vi "IMICSDK_GUI.vi"() -> ()   [LabVIEW 2011]
uses:
  <vilib>/Utility/cursorutil.llb/Set Cursor (Icon Pict).vi
panel:
  in  "Cluster":T1
  in  "resP":dbl=0.001
  in  "res":dbl=0.1
  in  "close at end":bool
  out "Status":T2(ring)
  in  "stop":bool
  in  "X":dbl(slide) min=0.0 scale=10.0..12.5
  in  "Y":dbl(slide) min=0.0 scale=0.0..22.0
  in  "Piezo":dbl(slide) step=0.005 scale=0.0..0.25 scale format="%#.4g"
  in  "Objektive":u16(ring) items=["Obj1 10x", "Obj2", "Obj3", "Obj4"]
  in  "FilterSchieber 1":u16(ring) items=["Filter 1", "Filter 2", "Filter 3"]
  in  "Z":dbl(slide) min=0.0 max=20.0 step=0.01 scale=18.0..20.0
  in  "handle":u64
  in  "comport":string="com1"
  # "xyz res."
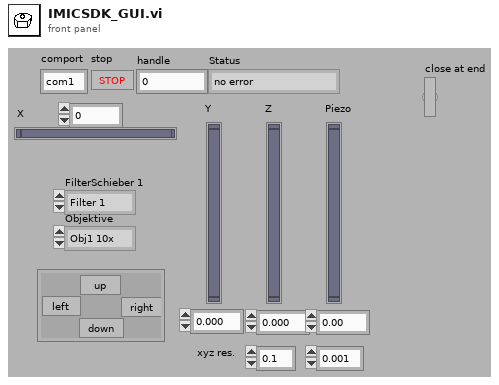
[diagram p1: front panel]
types:
  T1 = cluster{"up":bool, "left":bool, "right":bool, "down":bool}
  T2 = enum16{"no error", "missing axis", "missing Z axis", "missing Filter", "iMic not initialized", "no property", "wrong handle", "protocol not finished", "user parameter to long (>32 bits)", "no user parameter handle", "failed to open comport", "failed to initialize"}
  T3 = typedef "eventvkey.ctl" = enum16{"ASCII", "Enter", "Return", "Shift", "Ctrl", "Alt", "Cmd", "Opt", "Caps", "NumLock", "Clear", "Break", "Up", "Down", "Left", "Right", "Insert", "Delete", "Home", "End", "PageUp", "PageDown", "Escape", "Help", "Pause", "ScrollLock", "F1", "F2", "F3", "F4", "F5", "F6", "F7", "F8", "F9", "F10", "F11", "F12", "F13", "F14", "F15", "F16", "F17", "F18", "F19", "F20", "F21", "F22", "F23", "F24", "Play", "VolumeUp", "VolumeDown", "Mute", "Two Byte Char"}
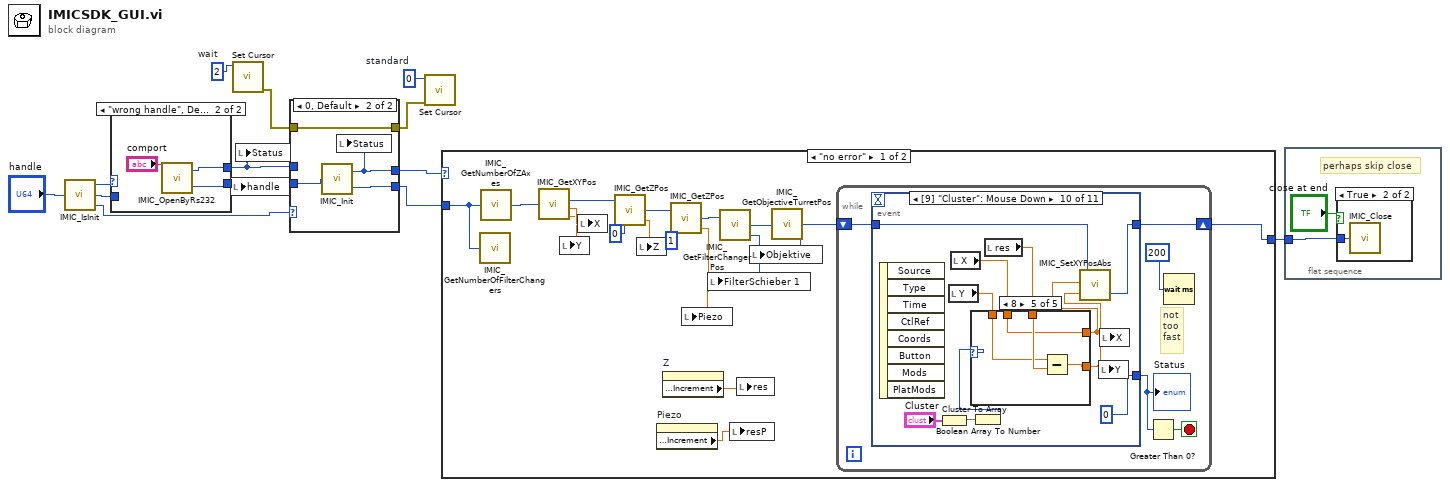
[diagram p0: block diagram]
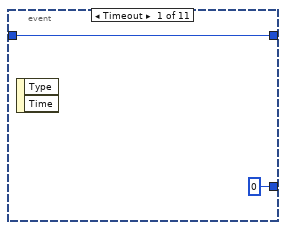
[diagram p5: hidden frame]
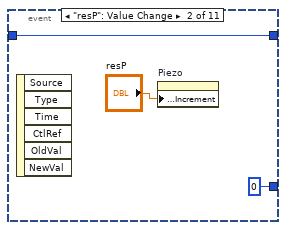
[diagram p6: hidden frame]
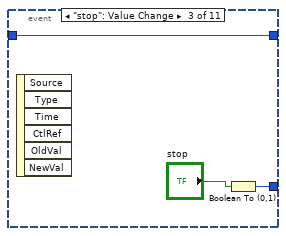
[diagram p7: hidden frame]
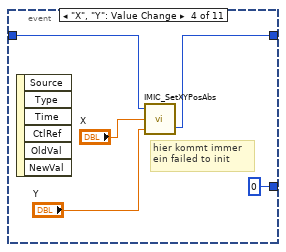
[diagram p8: hidden frame]
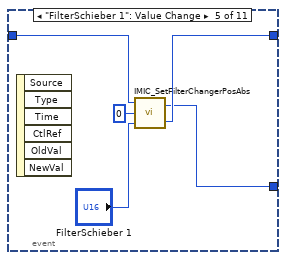
[diagram p9: hidden frame]
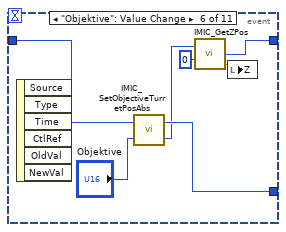
[diagram p10: hidden frame]
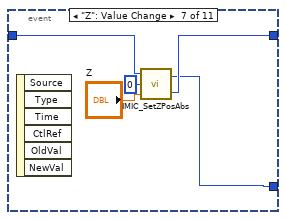
[diagram p11: hidden frame]
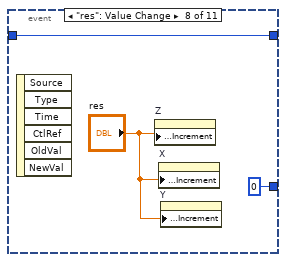
[diagram p12: hidden frame]
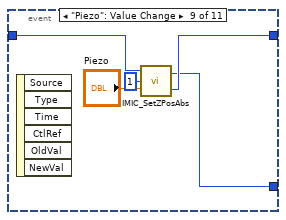
[diagram p13: hidden frame]
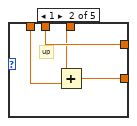
[diagram p15: hidden frame]
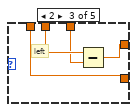
[diagram p16: hidden frame]
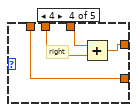
[diagram p17: hidden frame]
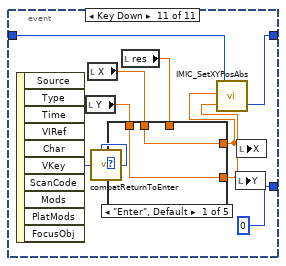
[diagram p18: hidden frame]
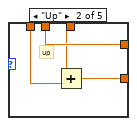
[diagram p19: hidden frame]
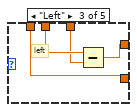
[diagram p20: hidden frame]
diagram:
  w8 = u16 2  # wait
  w9 = u16 0  # standard
  n1 = call "IMIC_IsInit.vi"("handle"="handle") -> ("output param"=w11:T2, "handle out"=w10:u64, "bool"=w3:i8)
  n2 = case shown="\"wrong handle\", Default" w11 {
    selector: w11 -> [w14 _]
    tunnel: [w15 w17] -> w2
    tunnel: w10 -> [w15 _]
    tunnel: [w14 w16] -> w1
    frame "no error" {
    }
    frame "wrong handle", Default {
      n3 = call "IMIC_OpenByRs232.vi"("comport"="comport") -> ("output param"=w16:T2, "handle out"=w17:u64)
    }
  }
  n4 = local write "handle"(w2) -> ()
  n5 = call-poly <vilib>:"Set Cursor.vi"("icon"=w8) -> ("error out"=w7:errorcluster)  [unwired: 9 in, 1 out]
  n6 = local write "Status"(w1) -> ()
  n7 = case shown="0, Default" w3 {
    tunnel: w7 -> [w19 w25]
    tunnel: [w19 w25] -> w6
    tunnel: w2 -> [w21 w24]
    tunnel: [w20 w22] -> w4
    tunnel: [w21 w23] -> w5
    tunnel: w1 -> [w20 _]
    frame 1 {
    }
    frame 0, Default {
      n8 = call "IMIC_Init.vi"("handle"=w24) -> ("output param"=w22:T2, "handle out"=w23:u64)
      n9 = local write "Status"(w22) -> ()
    }
  }
  n10 = call-poly <vilib>:"Set Cursor.vi"("error in (no error)"=w6, "icon"=w9) -> ()  [unwired: 8 in, 2 out]
  n11 = case shown="\"no error\"" w4 {
    tunnel: [w30 w144] -> w13
    tunnel: w5 -> [w29 w144]
    frame "no error" {
      n12 = call "IMIC_GetNumberOfFilterChangers.vi"("handle"=w29) -> ()  [unwired: 3 out]
      n13 = call "IMIC_GetNumberOfZAxes.vi"("handle"=w29) -> ("handle out"=w39:u64)  [unwired: 2 out]
      n14 = call "IMIC_GetXYPos.vi"("handle"=w39) -> ("handle out"=w35:u64, "xpos"=w37:dbl, "ypos"=w36:dbl)  [unwired: 1 out]
      n15 = local write "Y"(w36) -> ()
      n16 = local write "X"(w37) -> ()
      n17 = call "IMIC_GetZPos.vi"("handle"=w35, "index"=0) -> ("handle out"=w34:u64, "zpos"=w43:dbl)  [unwired: 1 out]
      n18 = local write "Z"(w43) -> ()
      n19 = property on="Piezo" class="Slide (strict)"() -> ("Data Entry Limits:Increment"=w27:dbl)  [unwired: 2 in, 2 out]
      n20 = property on="Z" class="Slide (strict)"() -> ("Data Entry Limits:Increment"=w28:dbl)  [unwired: 2 in, 2 out]
      n21 = call "IMIC_GetZPos.vi"("handle"=w34, "index"=1) -> ("handle out"=w33:u64, "zpos"=w26:dbl)  [unwired: 1 out]
      n22 = local write "Piezo"(w26) -> ()
      n23 = call "IMIC_GetFilterChangerPos.vi"("handle"=w33) -> ("handle out"=w32:u64, "Filter"=w42:i32)  [unwired: 1 in, 1 out]
      n24 = local write "FilterSchieber 1"(w42) -> ()
      n25 = local write "resP"(w27) -> ()
      n26 = local write "res"(w28) -> ()
      n27 = call "IMIC_GetObjectiveTurretPos.vi"("handle"=w32) -> ("handle out"=w31:u64, "Objective"=w41:i32)  [unwired: 1 out]
      n28 = local write "Objektive"(w41) -> ()
      n29 = while {
        shift-right: [w47] -> w30
        shift-left: w31 -> [w48]
        stop <- w44 stop-if-true
        # "not\ntoo\nfast"
        n30 = event shown="[9] \"Cluster\": Mouse Down" {
          selector: _ -> [_ _ _ _ _ _ _ _ _ _ _]
          dyn-events: _ -> [_ _ _ _ _ _ _ _ _ _ _]
          timeout: _ -> [_ _ _ _ _ _ _ _ _ _ _]
          tunnel: w48 -> [w50 w52 w56 w61 w64 w73 w76 w81 w85 w97 w125]
          tunnel: [w50 w52 w56 w60 w63 w68 w75 w81 w84 w88 w119] -> w47
          tunnel: [u16 0 ("output param") u16 0 ("output param") w54 u16 0 ("output param") w62 w71 w74 u16 0 ("output param") w83 0 0] -> w45
          event Timeout {
            n31 = event-data() -> ()  [unwired: 1 in, 2 out]
          }
          event "resP": Value Change {
            n32 = event-data() -> ()  [unwired: 1 in, 6 out]
            n33 = property on="Piezo" class="Slide (strict)"("Data Entry Limits:Increment"="resP") -> ()  [unwired: 2 in, 2 out]
          }
          event "stop": Value Change {
            n34 = event-data() -> ()  [unwired: 1 in, 6 out]
            n35 = Boolean To (0,1)(Boolean="stop") -> (0, 1=w54:i16)
          }
          event "X", "Y": Value Change {
            # "hier kommt immer\nein failed to init"
            n36 = event-data() -> ()  [unwired: 1 in, 6 out]
            n37 = call "IMIC_SetXYPosAbs.vi"("ypos"="Y", "xpos"="X", "handle"=w61) -> ("handle out"=w60:u64)  [unwired: 1 out]
          }
          event "FilterSchieber 1": Value Change {
            n38 = event-data() -> ()  [unwired: 1 in, 6 out]
            n39 = call "IMIC_SetFilterChangerPosAbs.vi"("Filter"="FilterSchieber 1", "index"=0, "handle"=w64) -> ("handle out"=w63:u64, "output param"=w62:T2)
          }
          event "Objektive": Value Change {
            n40 = event-data() -> ()  [unwired: 1 in, 6 out]
            n41 = call "IMIC_SetObjectiveTurretPosAbs.vi"("ObjectivePosAbs"="Objektive", "handle"=w73) -> ("handle out"=w69:u64, "output param"=w71:T2)
            n42 = call "IMIC_GetZPos.vi"("handle"=w69, "index"=0) -> ("handle out"=w68:u64, "zpos"=w67:dbl)  [unwired: 1 out]
            n43 = local write "Z"(w67) -> ()
          }
          event "Z": Value Change {
            n44 = event-data() -> ()  [unwired: 1 in, 6 out]
            n45 = call "IMIC_SetZPosAbs.vi"("zpos"="Z", "index"=0, "handle"=w76) -> ("handle out"=w75:u64, "output param"=w74:T2)
          }
          event "res": Value Change {
            n46 = event-data() -> ()  [unwired: 1 in, 6 out]
            n47 = property on="Z" class="Slide (strict)"("Data Entry Limits:Increment"="res") -> ()  [unwired: 2 in, 2 out]
            n48 = property on="X" class="Slide (strict)"("Data Entry Limits:Increment"="res") -> ()  [unwired: 2 in, 2 out]
            n49 = property on="Y" class="Slide (strict)"("Data Entry Limits:Increment"="res") -> ()  [unwired: 2 in, 2 out]
          }
          event "Piezo": Value Change {
            n50 = event-data() -> ()  [unwired: 1 in, 6 out]
            n51 = call "IMIC_SetZPosAbs.vi"("zpos"="Piezo", "index"=1, "handle"=w85) -> ("handle out"=w84:u64, "output param"=w83:T2)
          }
          event "Cluster": Mouse Down {
            n52 = event-data() -> ()  [unwired: 1 in, 8 out]
            n53 = Cluster To Array(cluster="Cluster") -> (array=w96:bool[])
            n54 = local read "Y"() -> (w91:dbl)
            n55 = local read "X"() -> (w92:dbl)
            n56 = Boolean Array To Number(Boolean array=w96) -> (number=w94:u32)
            n57 = local read "res"() -> (w93:dbl)
            n58 = case shown="8" w94 {
              tunnel: w93 -> [_ w101 w106 w110 w114]
              tunnel: w92 -> [w99 w103 w107 w109 w112]
              tunnel: w91 -> [w98 w102 w104 w108 w113]
              tunnel: [w99 w103 w105 w111 w112] -> w89
              tunnel: [w98 w100 w104 w108 w115] -> w90
              frame 0, Default {
              }
              frame 1 {
                # "up"
                n59 = Add(x=w101, y=w102) -> (x+y=w100:dbl)
              }
              frame 2 {
                # "left"
                n60 = Subtract(x=w107, y=w106) -> (x-y=w105:dbl)
              }
              frame 4 {
                # "right"
                n61 = Add(x=w110, y=w109) -> (x+y=w111:dbl)
              }
              frame 8 {
                n62 = Subtract(x=w113, y=w114) -> (x-y=w115:dbl)
              }
            }
            n63 = call "IMIC_SetXYPosAbs.vi"("ypos"=w90, "xpos"=w89, "handle"=w97) -> ("handle out"=w88:u64)  [unwired: 1 out]
            n64 = local write "Y"(w90) -> ()
            n65 = local write "X"(w89) -> ()
          }
          event Key Down {
            n66 = event-data() -> ("VKey"=w116:T3)  [unwired: 1 in, 9 out]
            n67 = local read "Y"() -> (w122:dbl)
            n68 = local read "X"() -> (w123:dbl)
            n69 = call <vilib>:"compatReturnToEnter.vi"("VKey"=w116) -> ("VKey"=w117:T3)
            n70 = local read "res"() -> (w124:dbl)
            n71 = case shown="\"Enter\", Default" w117 {
              tunnel: w124 -> [_ w129 w134 w138 w142]
              tunnel: w123 -> [w127 w131 w135 w137 w140]
              tunnel: w122 -> [w126 w130 w132 w136 w141]
              tunnel: [w127 w131 w133 w139 w140] -> w120
              tunnel: [w126 w128 w132 w136 w143] -> w121
              frame "Enter", Default {
              }
              frame "Up" {
                # "up"
                n72 = Add(x=w129, y=w130) -> (x+y=w128:dbl)
              }
              frame "Left" {
                # "left"
                n73 = Subtract(x=w135, y=w134) -> (x-y=w133:dbl)
              }
              frame "Right" {
                # "right"
                n74 = Add(x=w138, y=w137) -> (x+y=w139:dbl)
              }
              frame "Down" {
                n75 = Subtract(x=w141, y=w142) -> (x-y=w143:dbl)
              }
            }
            n76 = call "IMIC_SetXYPosAbs.vi"("ypos"=w121, "xpos"=w120, "handle"=w125) -> ("handle out"=w119:u64)  [unwired: 1 out]
            n77 = local write "Y"(w121) -> ()
            n78 = local write "X"(w120) -> ()
          }
        }
        "Status" <- w45
        n79 = Greater Than 0?(x=w45) -> (x > 0?=w44:bool)
        n80 = Wait (ms)(milliseconds to wait=u32 200) -> ()  [unwired: 1 out]
      }
    }
    frame "failed to open comport", Default {
    }
  }
  n81 = flat-sequence {
    tunnel: w13 -> [w146]
    frame #0 {
      # "perhaps skip close"
      n82 = case shown="True" "close at end" {
        tunnel: w146 -> [_ w147]
        frame False {
        }
        frame True {
          n83 = call "IMIC_Close.vi"("handle"=w147) -> ()  [unwired: 2 out]
        }
      }
    }
  }
